vi "AdjustCameraSettings.vi"(8 "error in (no error)":errorcluster, 9 "Contrast":dbl, 10 "Brightness":i64, 11 "Session In":T1) -> (0 "error out":errorcluster, 1 "ContrastWritable":bool, 2 "BrightnessWritable":bool, 3 "IMAQdx Session":T1)   [LabVIEW 2017]
uses:
  <vilib>/userdefined/High Color/IMAQdx.ctl
  <resource>/objmgr/imaqdx.rc
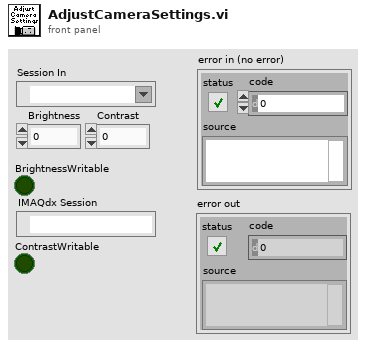
[diagram p1: front panel]
types:
  T1 = typedef "IMAQdx.ctl" = refnum<k21>
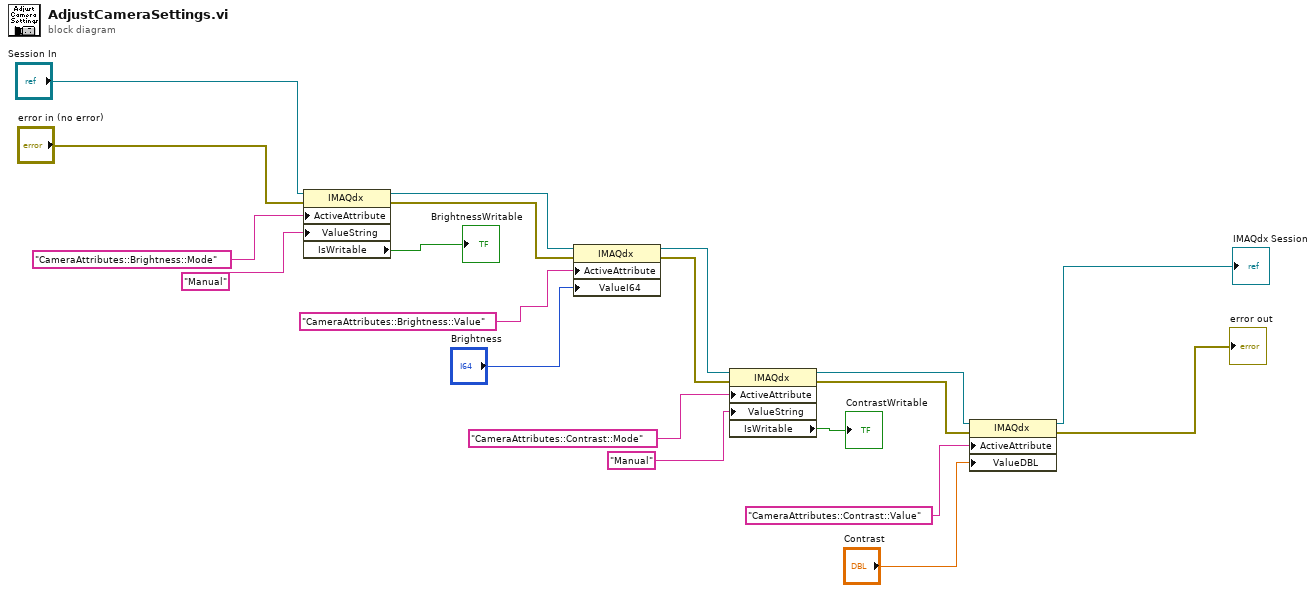
[diagram p0: block diagram]
diagram:
  n1 = property class="IMAQdx"(reference="Session In", error in="error in (no error)", "ActiveAttribute"="CameraAttributes::Brightness::Mode", "ValueString"="Manual") -> (reference out=w14:T1, error out=w13:errorcluster, "IsWritable"=→"BrightnessWritable":bool)
  n2 = property class="IMAQdx"(reference=w14, error in=w13, "ActiveAttribute"="CameraAttributes::Brightness::Value", "ValueI64"="Brightness") -> (reference out=w9:T1, error out=w8:errorcluster)
  n3 = property class="IMAQdx"(reference=w9, error in=w8, "ActiveAttribute"="CameraAttributes::Contrast::Mode", "ValueString"="Manual") -> (reference out=w4:T1, error out=w3:errorcluster, "IsWritable"=→"ContrastWritable":bool)
  n4 = property class="IMAQdx"(reference=w4, error in=w3, "ActiveAttribute"="CameraAttributes::Contrast::Value", "ValueDBL"="Contrast") -> (reference out=→"IMAQdx Session":T1, error out=→"error out":errorcluster)
